vi "Testar Controle.vi"(0 "Input":T1[](array[typedef]) {"height" format="%+4.3f"; "pixel_y" format="%+4.3f"; "pixel_x" format="%+4.3f"; "orientation" format="%+4.3f"; "y" format="%+4.3f"; "confidence" format="%4.3f"; "x" format="%+4.3f"}) -> ()   [LabVIEW 2016]
uses:
  SSL Detection Robot.ctl
panel:
  in  "Reinitialize":bool
  out "Position":dbl[](array[numeric])
  in  "Target":dbl[](array[numeric])
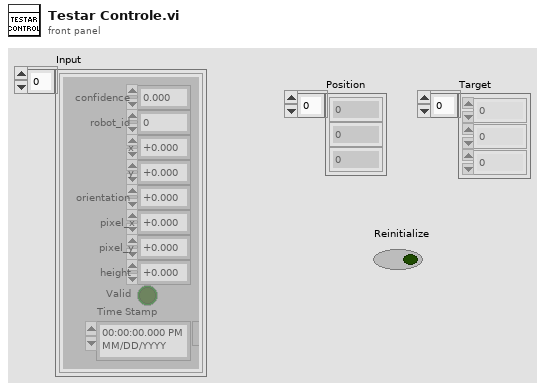
[diagram p1: front panel]
types:
  T1 = typedef "SSL Detection Robot.ctl" = cluster{"x":dbl, "robot_id":u32, "confidence":sgl, "y":sgl, "orientation":sgl, "pixel_x":sgl, "pixel_y":sgl, "height":sgl, "Valid":bool, "Time Stamp":timestamp}
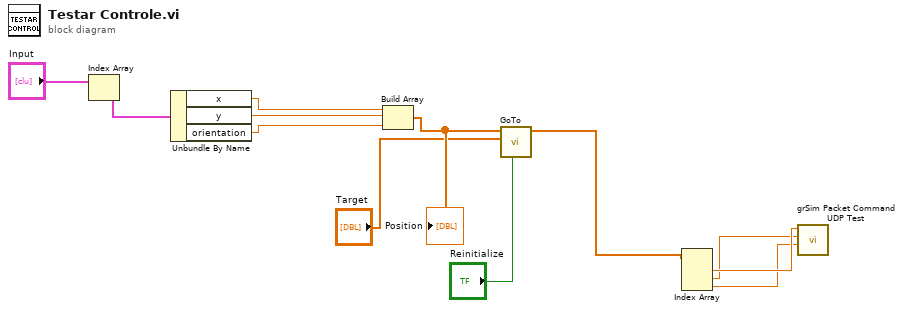
[diagram p0: block diagram]
diagram:
  n1 = Index Array(array="Input") -> (element=w11:T1)  [unwired: 1 in]
  n2 = Unbundle By Name(w11) -> ("x"=w10:dbl, "y"=w9:sgl, "orientation"=w8:sgl)
  n3 = Build Array(w10, w9, w8) -> (w7:dbl[])
  "Position" <- w7
  n4 = call "GoTo.vi"("Reinitialize"="Reinitialize", "Target"="Target", "Position"=w7) -> ("Output\nVelocity"=w5:dbl[])  [unwired: 8 in]
  n5 = Index Array(array=w5) -> (element #1=w4:dbl, element #2=w3:dbl, element #3=w1:dbl)  [unwired: 3 in]
  n6 = call "grSim Packet Command UDP Test.vi"("velangular"=w1, "velnormal"=w3, "veltangent"=w4) -> ()  [unwired: 9 in]
